vi "Current_Filepath.vi"(2 "Short_Name":string, 3 "Filename in":path, 4 "Data Type":string="Calibrations") -> (0 "Filename Out":path, 1 "Directory":path)   [LabVIEW 2020]
uses:
  Globals/Meas_global.vi
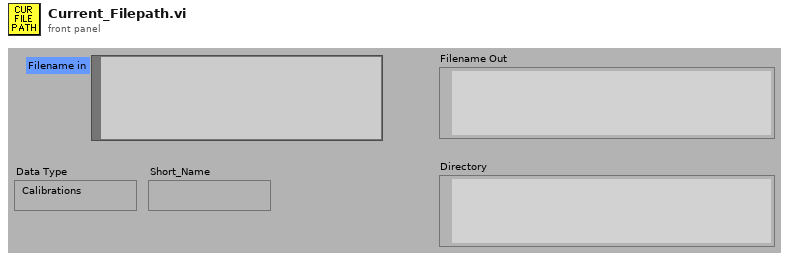
[diagram p1: front panel]
types:
  T1 = typedef "Post_Process.ctl" = enum16{"Take New Data", "Post Process Raw Data File"}
  T2 = cluster{"Filename in":path, "Data Type":string, "Short_Name":string}
  T3 = cluster{"Filename in":path, "Data Type":string, "Short_Name":string}[]
  T4 = cluster{"Filename in":path, "stripped path":path}
  T5 = cluster{"Filename in":path, "stripped path":path}[]
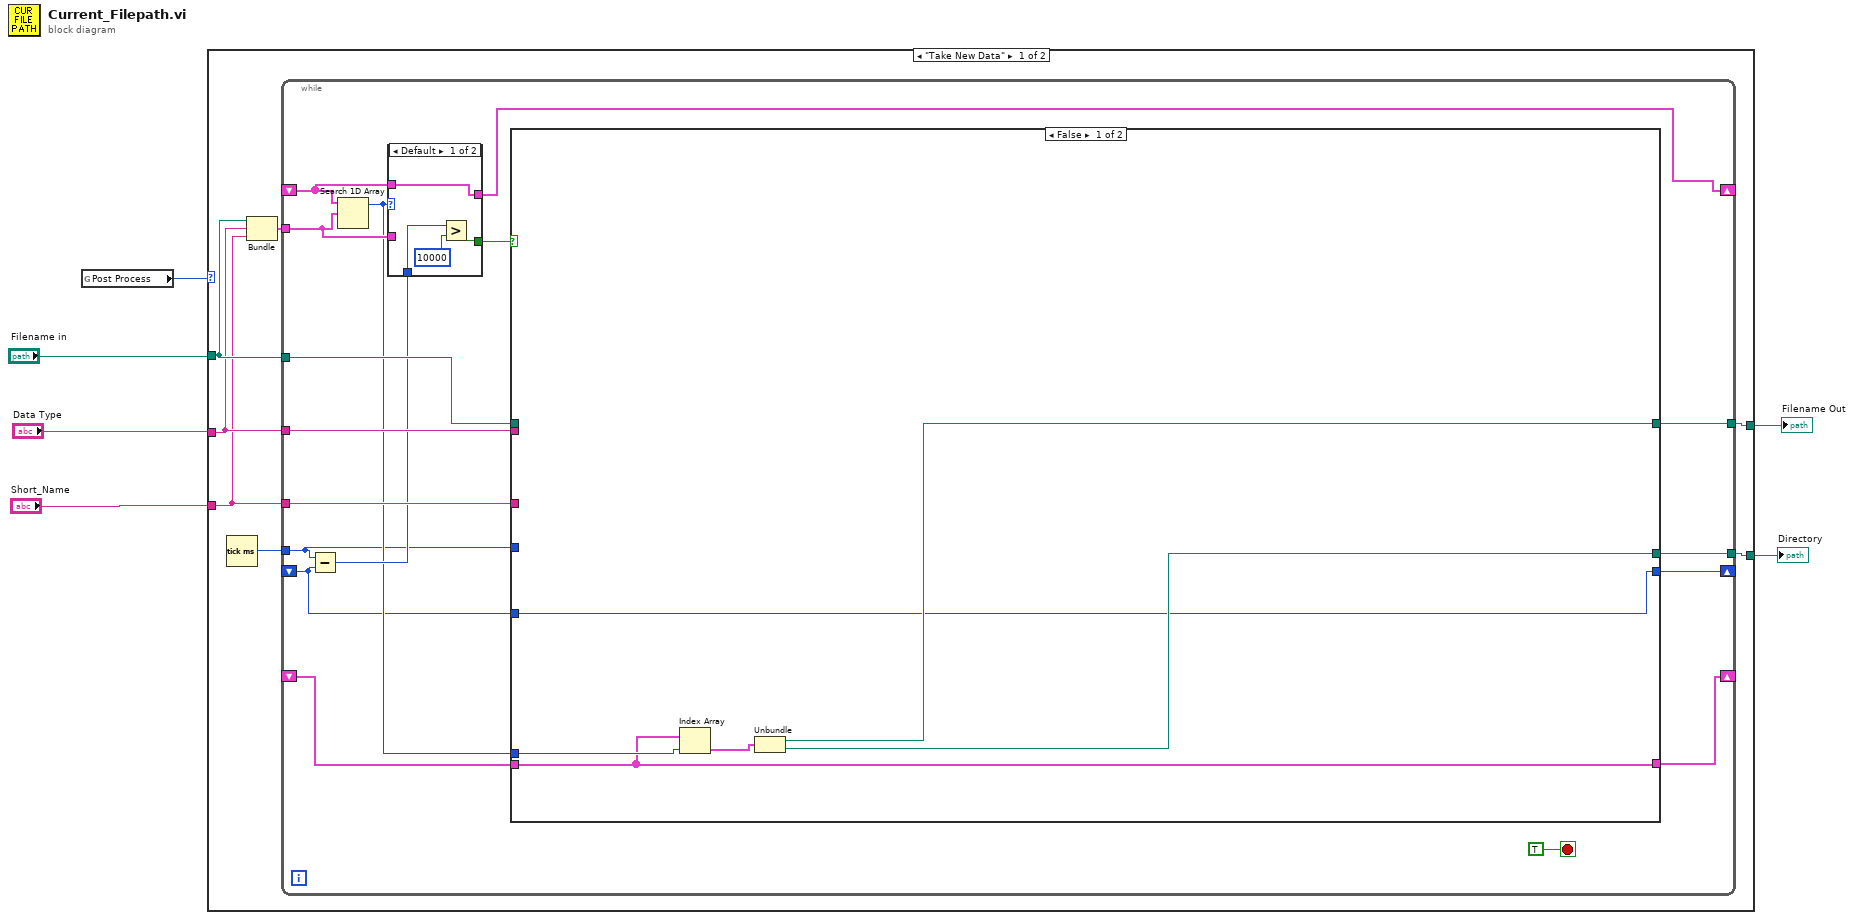
[diagram p0: block diagram]
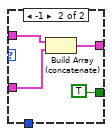
[diagram p2: hidden frame]
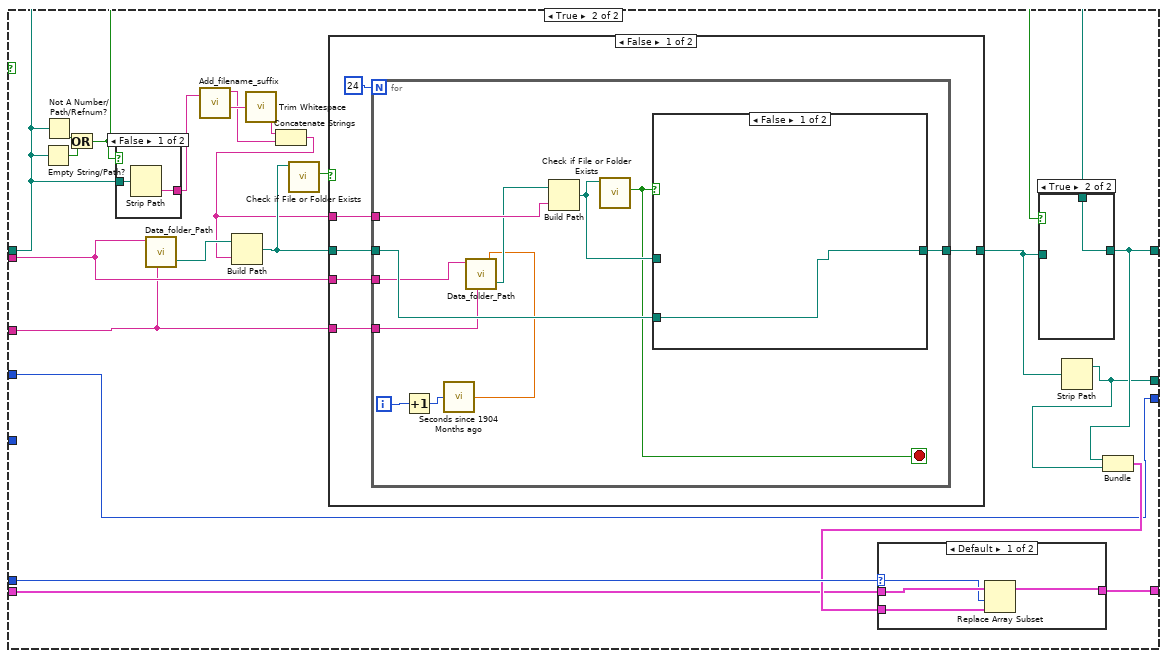
[diagram p3: hidden frame]
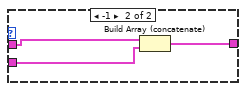
[diagram p4: hidden frame]
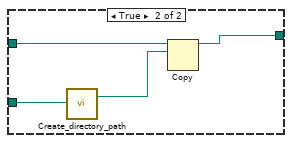
[diagram p5: hidden frame]
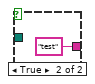
[diagram p8: hidden frame]
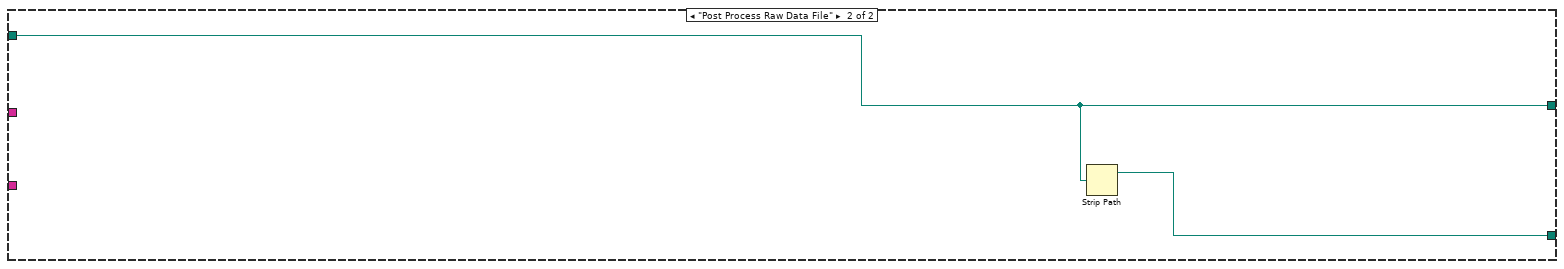
[diagram p9: hidden frame]
diagram:
  n1 = global read "Meas_global.vi" "Post Process"() -> (w3:T1)
  n2 = case shown="\"Take New Data\"" w3 {
    tunnel: "Filename in" -> [w11 w103]
    tunnel: "Data Type" -> [w10 _]
    tunnel: [w12 w103] -> w4
    tunnel: [w13 w102] -> w2
    tunnel: "Short_Name" -> [w9 _]
    frame "Take New Data" {
      n3 = Tick Count (ms)() -> (millisecond timer value=w7:u32)
      n4 = Bundle("Filename in"=w11, "Data Type"=w10, "Short_Name"=w9) -> (w8:T2)  [unwired: 1 in]
      n5 = while {
        tunnel: [w26] -> w13
        tunnel: w10 -> [w29]
        tunnel: w9 -> [w28]
        tunnel: [w27] -> w12
        tunnel: w11 -> [w30]
        shift-right: [w16] -> _
        shift-left: _ -> [w14]
        tunnel: w7 -> [w15]
        shift-right: [w22] -> _
        shift-left: _ -> [w24]
        tunnel: w8 -> [w23]
        shift-right: [w17] -> _
        shift-left: _ -> [w18]
        stop <- TRUE stop-if-true
        n6 = Subtract(x=w15, y=w14) -> (x-y=w20:u32)
        n7 = Search 1D Array(1D array=w24, element=w23) -> (index of element=w19:i32)  [unwired: 1 out]
        n8 = case shown="Default" w19 {
          tunnel: w24 -> [w34 w38]
          tunnel: w23 -> [_ w37]
          tunnel: [w34 w36] -> w22
          tunnel: [w32 TRUE] -> w21
          tunnel: w20 -> [w33 _]
          frame Default {
            n9 = Greater?(x=w33, y=u32 10000) -> (0:w32:bool)
          }
          frame -1 {
            n10 = Build Array (concatenate)(w38, w37) -> (w36:T3)
          }
        }
        n11 = case shown="False" w21 {
          tunnel: [w41 w49] -> w26
          tunnel: w29 -> [_ w63]
          tunnel: w28 -> [_ w61]
          tunnel: [w42 w51] -> w27
          tunnel: w30 -> [_ w53]
          tunnel: w19 -> [w44 w52]
          tunnel: w18 -> [w40 w47]
          tunnel: [w40 w46] -> w17
          tunnel: [w39 w45] -> w16
          tunnel: w15 -> [_ w45]
          tunnel: w14 -> [w39 _]
          frame False {
            n12 = Index Array(array=w40, index=w44) -> (element=w43:T4)
            n13 = Unbundle(w43) -> ("Filename in"=w42:path, "stripped path"=w41:path)
          }
          frame True {
            n14 = Empty String/Path?(string/path=w53) -> (empty?=w65:bool)
            n15 = Not A Number/Path/Refnum?(number/path/refnum=w53) -> (NaN/Path/Refnum?=w66:bool)
            n16 = Or(x=w66, y=w65) -> (x .or. y?=w64:bool)
            n17 = case shown="False" w64 {
              tunnel: [w100 "test" ("name")] -> w58
              tunnel: w53 -> [w99 _]
              frame False {
                n18 = Strip Path(path=w99) -> (name=w100:string)  [unwired: 1 out]
              }
              frame True {
              }
            }
            n19 = call "Data_folder_Path.vi"("Data Type"=w63, "Short_Name"=w61) -> ("Data Folder"=w62:path)  [unwired: 4 in]
            n20 = call "Add_filename_suffix.vi"("Filename"=w58) -> ("Original Suffix"=w55:string, "Base name"=w57:string)  [unwired: 1 in, 2 out]
            n21 = call <vilib>:"Trim Whitespace.vi"("string"=w57) -> ("trimmed string"=w56:string)  [unwired: 1 in]
            n22 = Concatenate Strings(w56, w55) -> (w54:string)
            n23 = Build Path(base path=w62, name or relative path=w54) -> (appended path=w60:path)
            n24 = call <vilib>:"Check if File or Folder Exists.vi"("path"=w60) -> ("file or folder exists?"=w59:bool)  [unwired: 1 in, 9 out]
            n25 = case shown="False" w59 {
              tunnel: [w79 w96] -> w50
              tunnel: w63 -> [w77 _]
              tunnel: w54 -> [w76 _]
              tunnel: w60 -> [w75 w96]
              tunnel: w61 -> [w74 _]
              frame False {
                n26 = for {
                  N: 24 -> [_]
                  tunnel: w76 -> [w90]
                  tunnel: w77 -> [w88]
                  tunnel: w74 -> [w86]
                  tunnel: w75 -> [w89]
                  tunnel: [w87] -> w79
                  i -> [w85]
                  stop <- w81 stop-if-true
                  n27 = Increment(x=w85) -> (x+1=w80:i32)
                  n28 = call "Seconds since 1904 Months ago.vi"("No of Months ago"=w80) -> ("Seconds since 1904"=w82:dbl)
                  n29 = call "Data_folder_Path.vi"("Data Type"=w88, "Short_Name"=w86, "seconds"=w82) -> ("Data Folder"=w83:path)  [unwired: 3 in]
                  n30 = Build Path(base path=w83, name or relative path=w90) -> (appended path=w84:path)
                  n31 = call <vilib>:"Check if File or Folder Exists.vi"("path"=w84) -> ("file or folder exists?"=w81:bool)  [unwired: 1 in, 9 out]
                  n32 = case shown="False" w81 {
                    tunnel: w84 -> [_ w95]
                    tunnel: w89 -> [w91 w93]
                    tunnel: [w91 w94] -> w87
                    frame False {
                    }
                    frame True {
                      n33 = call "Create_directory_path.vi"("Path name"=w93) -> ("Path name Out"=w92:path)  [unwired: 2 in, 1 out]
                      n34 = Copy(10:w92, 11:w95) -> (3:w94:path)  [unwired: 3 in, 2 out]
                    }
                  }
                }
              }
              frame True {
              }
            }
            n35 = case shown="True" w64 {
              tunnel: w50 -> [w97 _]
              tunnel: [w97 w98] -> w51
              tunnel: w53 -> [_ w98]
              frame False {
              }
              frame True {
              }
            }
            n36 = Strip Path(path=w50) -> (stripped path=w49:path)  [unwired: 1 out]
            n37 = Bundle("Filename in"=w51, "stripped path"=w49) -> (w48:T4)  [unwired: 1 in]
            n38 = case shown="Default" w52 {
              selector: w52 -> [w68 _]
              tunnel: w48 -> [w69 w73]
              tunnel: w47 -> [w70 w72]
              tunnel: [w67 w71] -> w46
              frame Default {
                n39 = Replace Array Subset(array=w70, new element=w69, index=w68) -> (w67:T5)
              }
              frame -1 {
                n40 = Build Array (concatenate)(w72, w73) -> (w71:T5)
              }
            }
          }
        }
      }
    }
    frame "Post Process Raw Data File" {
      n41 = Strip Path(path=w103) -> (stripped path=w102:path)  [unwired: 1 out]
    }
  }
  "Filename Out" <- w4
  "Directory" <- w2
